vi "image_to_ui_conversion.vi"() -> ()   [LabVIEW 2020]
uses:
  src/models/llm_openai_chatmodels/llm_openai_chatmodels.lvclass
  D:/AI/labview-llm-libraries/src/models/abstract_llm_base/abstract_llm_base.lvclass
  src/models/llm_gemini_chatmodels/llm_gemini_chatmodels.lvclass
  src/models/message_image/message_image.lvclass
  D:/AI/labview-llm-libraries/src/models/abstract_message_base/abstract_message_base.lvclass
  src/models/message_text/message_text.lvclass
  src/models/llm_openai_chatmodels/Instantiate_llm_openai.vi
  src/models/llm_gemini_chatmodels/Instantiate_llm_gemini.vi
  src/models/message_image/create_image_message.vi
  src/models/message_text/create_text_message.vi
  src/models/message_text/get_text_message_value.vi
  src/models/abstract_llm_base/abstract_llm_base.lvclass
  src/models/abstract_llm_chatcompletion/abstract_llm_chatcompletion.lvclass
panel:
  out "Status of UI creation":string
  out "Model Generated JSON string":string
  out "User Given Image":picture
  in  "Input Image":path
  in  "Provider Selector":enum32{"OpenAI", "Gemini"}(tab)
  in  "model_name":string(combo)="gpt-4o-mini"
  out "openai_key":string
  in  "model_name":string(combo)="gemini-2.0-flash"
  out "Gemini_api_key":string
  out "error out":errorcluster
  # "1. Ensure you assign the OpenAI Key to environmental variables so it is away from the code and easy to use the examples in future.\n\n2. Use the \"Set_Env_Var.vi\" from examples/utils folder to set the key \"labview_llm_openai_key\"."
  # "1. Ensure you assign the Gemini API Key to environmental variables so it is away from the code and easy to use the examples in future.\n\n2. Use the \"Set_Env_Var.vi\" from examples/utils folder to set the key \"labview_llm_gemini_key\"."
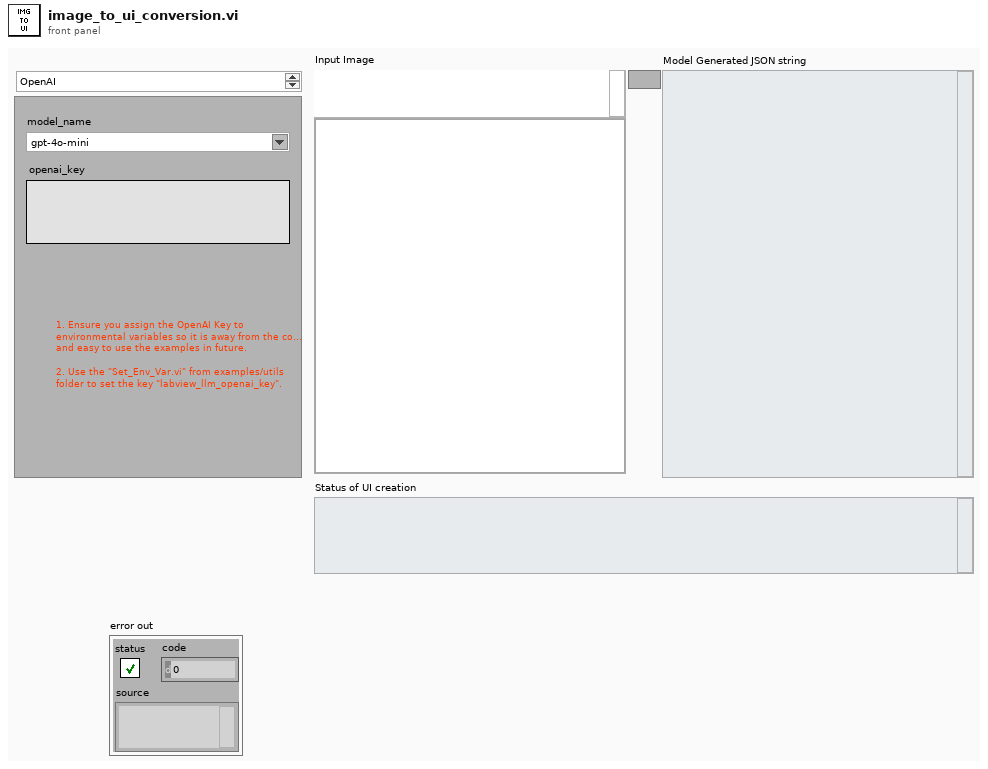
[diagram p1: front panel]
types:
  T1 = typedef "imagedata.ctl" = cluster{"image type":i32, "image depth":i32, "image":u8[], "mask":u8[], "colors":u32[], "Rectangle":cluster{"left":i16, "top":i16, "right":i16, "bottom":i16}}
  T2 = typedef "LVBoundsTypeDef.ctl" = cluster{"Width":u32, "Height":u32}
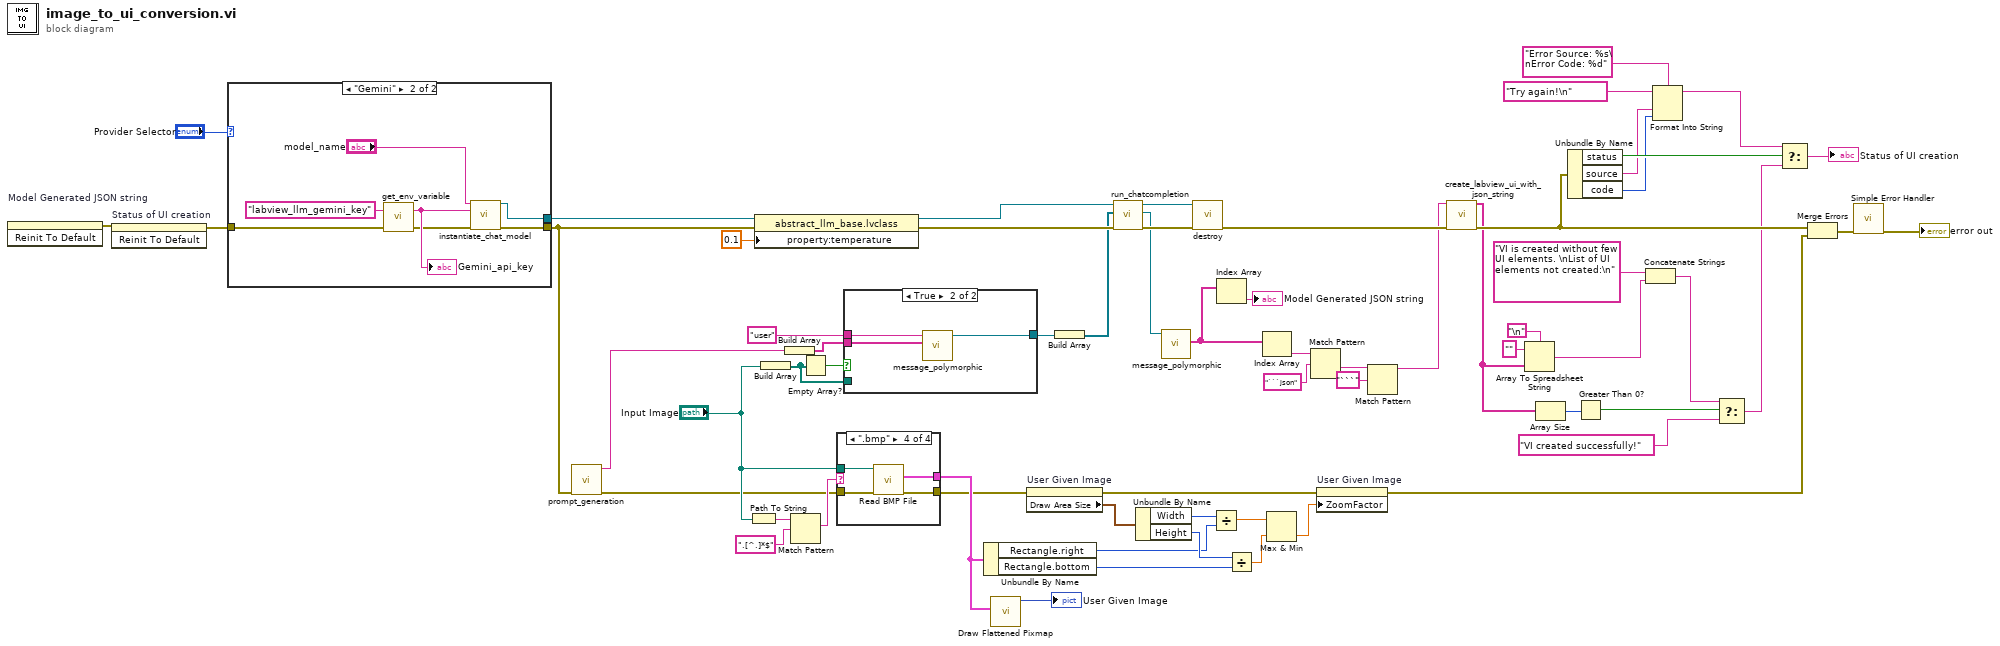
[diagram p0: block diagram]
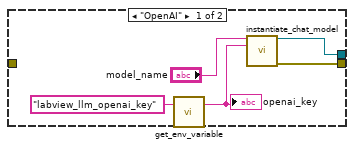
[diagram p2: hidden frame]
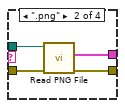
[diagram p4: hidden frame]
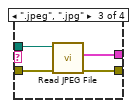
[diagram p5: hidden frame]
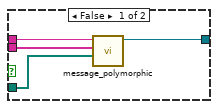
[diagram p6: hidden frame]
diagram:
  n1 = invoke on="Model Generated JSON string" class="Str" method="Reinit To Default"() -> (error out=w11:errorcluster)  [unwired: 3 in, 2 out]
  n2 = invoke on="Status of UI creation" class="Str" method="Reinit To Default"(error in=w11) -> (error out=w12:errorcluster)  [unwired: 2 in, 2 out]
  n3 = case shown="\"Gemini\"" "Provider Selector" {
    tunnel: [w68 w74] -> w18
    tunnel: [w67 w75] -> w46
    tunnel: w12 -> [_ w70]
    frame "OpenAI" {
      n4 = call "get_env_variable.vi"("Environment Variable Name"="labview_llm_openai_key") -> ("Value"=w65:string)  [unwired: 1 in, 1 out]
      "openai_key" <- w65
      n5 = call-poly "instantiate_chat_model.vi"("model_name"="model_name", "openai_key"=w65) -> ("llm_openai out"=w67:refnum<class "llm_openai_chatmodels.lvclass">, "error out"=w68:errorcluster)  [unwired: 12 in]
    }
    frame "Gemini" {
      n6 = call "get_env_variable.vi"("Environment Variable Name"="labview_llm_gemini_key") -> ("Value"=w71:string)  [unwired: 1 in, 1 out]
      "Gemini_api_key" <- w71
      n7 = call-poly "instantiate_chat_model.vi"("model_name"="model_name", "Gemini_api_key"=w71, "error in (no error)"=w70) -> ("llm_openai out"=w75:refnum<class "llm_gemini_chatmodels.lvclass">, "error out"=w74:errorcluster)  [unwired: 11 in]
    }
  }
  n8 = call "prompt_generation.vi"("error in (no error)"=w18) -> ("error out"=w19:errorcluster, "prompt"=w20:string)  [unwired: 9 in]
  n9 = Path To String(path="Input Image") -> (string=w22:string)
  n10 = property class="abstract_llm_base.lvclass"(reference=w46, error in=w18, "property:temperature"=0.1 ("temperature")) -> (reference out=w64:refnum<class "abstract_llm_base.lvclass">, error out=w63:errorcluster)
  n11 = Build Array("Input Image") -> (w58:path[])
  n12 = Build Array(w20) -> (w60:string[])
  n13 = Match Pattern(string=w22, regular expression=".[^.]*$") -> (match substring=w21:string)  [unwired: 1 in, 3 out]
  n14 = Empty Array?(array=w58) -> (empty?=w59:bool)
  n15 = case shown="\".bmp\"" w21 {
    tunnel: [_ w80 w81 w85] -> w43
    tunnel: [w76 w79 w83 w87] -> w31
    tunnel: w19 -> [w76 w78 w84 w88]
    tunnel: "Input Image" -> [_ w77 w82 w86]
    frame Default {
    }
    frame ".png" {
      n16 = call <vilib>:"Read PNG File.vi"("error in (no error)"=w78, "path to PNG file"=w77) -> ("error out"=w79:errorcluster, "image data"=w80:T1)  [unwired: 7 in, 1 out]
    }
    frame ".jpeg", ".jpg" {
      n17 = call <vilib>:"Read JPEG File.vi"("error in (no error)"=w84, "path to JPEG file"=w82) -> ("error out"=w83:errorcluster, "image data"=w81:T1)  [unwired: 7 in, 1 out]
    }
    frame ".bmp" {
      n18 = call <vilib>:"Read BMP File.vi"("error in (no error)"=w88, "path to BMP file"=w86) -> ("error out"=w87:errorcluster, "image data"=w85:T1)  [unwired: 7 in, 1 out]
    }
  }
  n19 = case shown="True" w59 {
    tunnel: w60 -> [w92 w95]
    tunnel: [w91 w94] -> w56
    tunnel: w58 -> [w89 _]
    tunnel: "user" ("role") -> [w90 w93]
    frame False {
      n20 = call-poly "message_polymorphic.vi"("images"=w89, "text"=w92, "role"=w90) -> ("message_text out"=w91:refnum<class "message_image.lvclass">)  [unwired: 7 in, 1 out]
    }
    frame True {
      n21 = call-poly "message_polymorphic.vi"("content"=w95, "role"=w93) -> ("message_text out"=w94:refnum<class "message_text.lvclass">)  [unwired: 8 in, 1 out]
    }
  }
  n22 = Unbundle By Name(w43) -> ("Rectangle.right"=w39:i16, "Rectangle.bottom"=w40:i16)
  n23 = call <vilib>:"Draw Flattened Pixmap.vi"("image data"=w43) -> ("new picture"=→"User Given Image":picture)  [unwired: 8 in]
  n24 = property on="User Given Image" class="Pict"(error in=w31) -> (error out=w32:errorcluster, "Draw Area Size"=w42:T2)  [unwired: 1 in, 1 out]
  n25 = Build Array(w56) -> (w55:refnum<class "abstract_message_base.lvclass">[])
  n26 = call "run_chatcompletion.vi"("error in (no error)"=w63, "Messages"=w55, "abstract_llm_chatcompletion in"=w64) -> ("error out"=w62:errorcluster, "Response"=w54:refnum<class "abstract_message_base.lvclass">, "abstract_llm_chatcompletion out"=w61:refnum<class "abstract_llm_base.lvclass">)  [unwired: 6 in]
  n27 = Unbundle By Name(w42) -> ("Width"=w38:u32, "Height"=w41:u32)
  n28 = call-poly "message_polymorphic.vi"("abstract_message_base.lvclass"=w54) -> ("content"=w34:string[])  [unwired: 8 in, 2 out]
  n29 = call-dynamic "destroy.vi"("error in (no error)"=w62, "abstract_llm_base in"=w61) -> ("error out"=w49:errorcluster)  [unwired: 8 in, 1 out]
  n30 = Divide(x=w38, y=w39) -> (x/y=w37:dbl)
  n31 = Index Array(array=w34) -> (element=→"Model Generated JSON string":string)  [unwired: 1 in]
  n32 = Divide(x=w41, y=w40) -> (x/y=w36:dbl)
  n33 = Index Array(array=w34) -> (element=w53:string)  [unwired: 1 in]
  n34 = Max & Min(x=w37, y=w36) -> (min(x,y)=w35:dbl)  [unwired: 1 out]
  n35 = Match Pattern(string=w53, regular expression="```json") -> (after substring=w51:string)  [unwired: 1 in, 3 out]
  n36 = property on="User Given Image" class="Pict"(error in=w32, "ZoomFactor"=w35) -> (error out=w28:errorcluster)  [unwired: 1 in, 1 out]
  n37 = Match Pattern(string=w51, regular expression="```") -> (before substring=w48:string)  [unwired: 1 in, 3 out]
  n38 = call "create_labview_ui_with_json_string.vi"("json string"=w48, "error in (no error)"=w49) -> ("not created ui objects"=w7:string[], "error out"=w27:errorcluster)  [unwired: 12 in]
  n39 = Array To Spreadsheet String(delimiter (Tab)="\n", array=w7, 3:"" ("format string")) -> (spreadsheet string=w4:string)
  n40 = Array Size(array=w7) -> (size(s)=w10:i32)
  n41 = Unbundle By Name(w27) -> ("status"=w26:bool, "source"=w15:string, "code"=w14:i32)
  n42 = Greater Than 0?(x=w10) -> (x > 0?=w9:bool)
  n43 = Concatenate Strings("VI is created without few UI elements. \nList of UI elements not created:\n", w4) -> (w3:string)
  n44 = Format Into String(format string="Error Source: %s\nError Code: %d", initial string="Try again!\n" ("t"), w15, w14) -> (resulting string=w13:string)  [unwired: 1 in, 1 out]
  n45 = Select(t=w3, s=w9, f="VI created successfully!") -> (s? t:f=w2:string)
  n46 = Select(t=w13, s=w26, f=w2) -> (s? t:f=→"Status of UI creation":string)
  n47 = Merge Errors(w27, w28) -> (w29:errorcluster)
  n48 = call <vilib>:"Simple Error Handler.vi"("error in (no error)"=w29) -> ("error out"=→"error out":errorcluster)  [unwired: 4 in, 4 out]
